vi "SP Convert X-Y to Points.vi"(9 "Frequency":dbl[](array[numeric]), 10 "X-Y":cluster{"x values":dbl[], "y values":dbl[]}[](array[cluster])) -> (2 "X-Y Points":cluster{"x values":dbl[], "y values":dbl[]}[](array[cluster]))   [LabVIEW 2011]
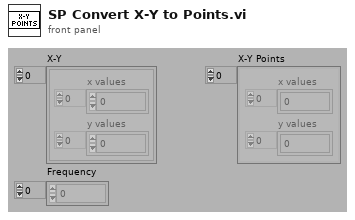
[diagram p1: front panel]
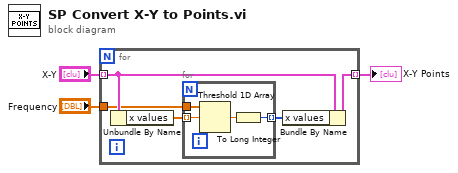
[diagram p0: block diagram]
diagram:
  n1 = for {
    tunnel: "X-Y" -> [w8] mode=indexing
    tunnel: "Frequency" -> [w7]
    tunnel: [w4] -> w1 mode=indexing
    n2 = Unbundle By Name(w8) -> ("x values"=w6:dbl[])
    n3 = for {
      tunnel: w7 -> [w12]
      tunnel: w6 -> [w11] mode=indexing
      tunnel: [w9] -> w5 mode=indexing
      n4 = Threshold 1D Array(2:w11, 3:w12) -> (0:w10:dbl)  [unwired: 1 out]
      n5 = To Long Integer(number=w10) -> (32bit integer=w9:i32)
    }
    n6 = Bundle By Name(cluster=w8, "x values"=w5) -> (w4:cluster{"x values":dbl[], "y values":dbl[]})
  }
  "X-Y Points" <- w1
